vi "Download Temporary GPack.vi"(8 "error in (no error)":errorcluster, 11 "NamedPackage in":refnum<class "NamedPackage.lvclass">) -> (0 "error out":errorcluster, 3 "NamedPackage out":refnum<class "NamedPackage.lvclass">)   [LabVIEW 2020, in "GPack.lvlib" / "NamedPackage.lvclass"]
uses:
  NamedPackage.lvclass
  NamedPackage.lvclass/NamedPackage.ctl
  GPack File/GPack File.lvclass
  <vilib>/Utility/sysdir.llb/System Directory Type.ctl
  GPack.lvlib
  <vilib>/httpClient/LabVIEWHTTPClient.lvlib
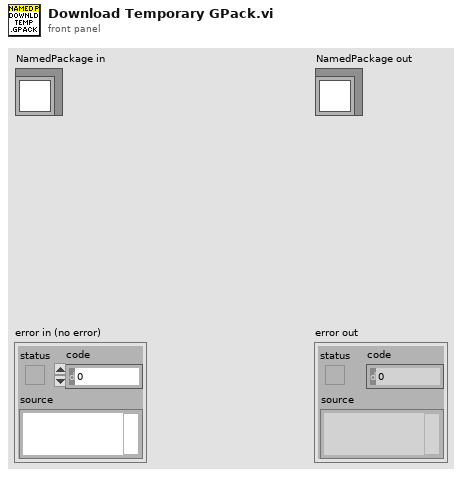
[diagram p1: front panel]
types:
  T1 = typedef "System Directory Type.ctl" = i32
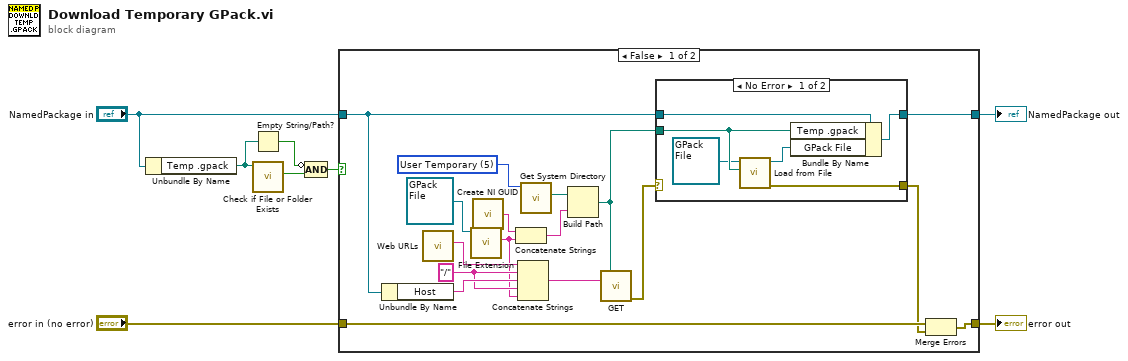
[diagram p0: block diagram]
diagram:
  n1 = Unbundle By Name("NamedPackage in") -> ("Temp .gpack"=w3:path)
  n2 = Empty String/Path?(string/path=w3) -> (empty?=w1:bool)
  n3 = call <vilib>:"Check if File or Folder Exists.vi"("path"=w3) -> ("file or folder exists?"=w4:bool)  [unwired: 8 in, 2 out]
  n4 = Compound Arithmetic op=AND(invert w1, w4) -> (w2:bool)
  n5 = case shown="False" w2 {
    tunnel: "error in (no error)" -> [w24 w35]
    tunnel: [w13 w34] -> w7
    tunnel: [w12 w35] -> w6
    tunnel: "NamedPackage in" -> [w11 w34]
    frame False {
      w19 = T1 5 items=["User Home"=0, "User Desktop"=1, "User Documents"=2, "User Application Data"=3, "User Preferences"=4, "User Temporary"=5, "Public Documents"=6, "Public Application Data"=7, "Public Preferences"=8, "Public Cache"=13, "System Core Libraries"=9, "System Installed Libraries"=10, "Application Files"=11, "Boot Volume Root"=12] ("system directory type")
      w16 = "/" ("string")
      n6 = Unbundle By Name(w11) -> ("Host"=w22:string)
      n7 = call "Web URLs.vi"() -> ("Index"=w23:string)  [unwired: 10 in, 1 out]
      n8 = call-dynamic "File Extension.vi"("GPack File in"=refnum<class "GPack File.lvclass"> refnum) -> ("File Extension"=w15:string)  [unwired: 9 in, 1 out]
      n9 = call <vilib>:"Create NI GUID.vi"() -> ("NI GUID"=w21:string)
      n10 = Concatenate Strings(w21, w15) -> (w17:string)
      n11 = Concatenate Strings(w23, w16, w22, w16, w15) -> (w14:string)
      n12 = call <vilib>:"Get System Directory.vi"("system directory type"=w19) -> ("system directory"=w18:path)  [unwired: 10 in]
      n13 = Build Path(base path=w18, name or relative path=w17) -> (appended path=w9:path)
      n14 = call <vilib>:"GET.vi"("output file"=w9, "url"=w14) -> ("error out"=w25:errorcluster)  [unwired: 10 in, 3 out]
      n15 = case shown="No Error" w25 {
        selector: w25 -> [_ w32]
        tunnel: w11 -> [w31 w33]
        tunnel: [w30 w33] -> w13
        tunnel: w9 -> [w29 _]
        tunnel: [w26 w32] -> w10
        frame No Error {
          n16 = call-dynamic "Load from File.vi"("Path"=w29, "GPack File in"=refnum<class "GPack File.lvclass"> refnum) -> ("error out"=w26:errorcluster, "GPack File out"=w27:refnum<class "GPack File.lvclass">)  [unwired: 8 in]
          n17 = Bundle By Name(cluster=w31, "Temp .gpack"=w29, "GPack File"=w27) -> (w30:refnum<class "NamedPackage.lvclass">)
        }
        frame Error {
        }
      }
      n18 = Merge Errors(w24, w10) -> (w12:errorcluster)
    }
    frame True {
      # "Already downloaded, do nothing."
    }
  }
  "error out" <- w6
  "NamedPackage out" <- w7
